vi "Adquisicion Sonido Continuo pruebas.vi"() -> ()   [LabVIEW 2023]
uses:
  <vilib>/sound2/lvsound2.llb/Sound Data Format.ctl
  <vilib>/sound2/lvsound2.llb/Sampling Mode.ctl
  <vilib>/sound2/lvsound2.llb/Sound Input Read (DBL).vi
  <vilib>/Analysis/3filter.llb/Butterworth Filter (DBL).vi
  <vilib>/measure/mamon.llb/Waveform Peak Detection for 1 Chan.vi
  <vilib>/measure/maspectr.llb/FFT Power Spectrum and PSD for 1 Chan.vi
  <vilib>/Waveform/DWDTOps.llb/DWDT Analog to Digital.vi
  <vilib>/express/express analysis/Spectral/Block/exnSpectralBlock spectral measurements power poly.vi
  <vilib>/express/express analysis/Spectral/Block/exnSpectralBlock spectral measurements power array WFM.vi
  <vilib>/express/express analysis/Spectral/XNode/ExpressSpectralMeasurementsBlockNode.xnode
  <vilib>/measure/NI_MABase.lvlib
  <vilib>/measure/NI_MAPro.lvlib
  <vilib>/Analysis/NI_AALBase.lvlib
panel:
  in  "Phase 6":dbl(knob) scale=0.0..360.0
  in  "alta frec filtrada 2":T1(ring)
  in  "phase 5":dbl(knob) scale=0.0..360.0
  in  "baja frec filtrada 2":T1(ring)
  in  "frequency 2":dbl=10.0 format="%0.2p"
  in  "frequency":dbl=10.0 format="%0.2p"
  out "# found":i32
  in  "peaks/valleys":u16(ring) items=["Peaks", "Valleys"]
  out "Lissajous 2":cluster{"Array":dbl[], "Array":dbl[]}(graph)
  in  "señal alta frec filtrada":T1(ring)
  in  "phase 4":dbl format="%.2p"
  in  "phase 3":dbl
  in  "señal baja frec filtrada":T1(ring)
  in  "alpha":dbl
  in  "stop 2":bool
  out "Lissajous":cluster{"Array":dbl[], "Array":dbl[]}[](graph)
  in  "señal alta frec":T1(ring)
  in  "phase 2":dbl format="%.2p"
  in  "Señal baja frec":T1(ring)
  in  "phase":dbl
  out "Max banda 2":i32
  out "Max banda 1":i32
  out "Tamaño banda 2":i32
  out "Plano Y":dbl[](array[numeric])
  out "Tamaño banda 1":i32
  out "Plano X":dbl[](array[numeric])
  in  "banda 2":dbl
  in  "banda 1":dbl
  out "Tamaño Señal":i32
  out "Espectro Señal":cluster{"f0":dbl, "df":dbl, "magnitude":dbl[]}[](graph)
  in  "stop":bool
  in  "Tiempo de refresco":dbl
  out "Señal Adquirida":waveform(dbl)[](graph)
  # "Señal sin Filtrado"
  # "Señal Filtrada"
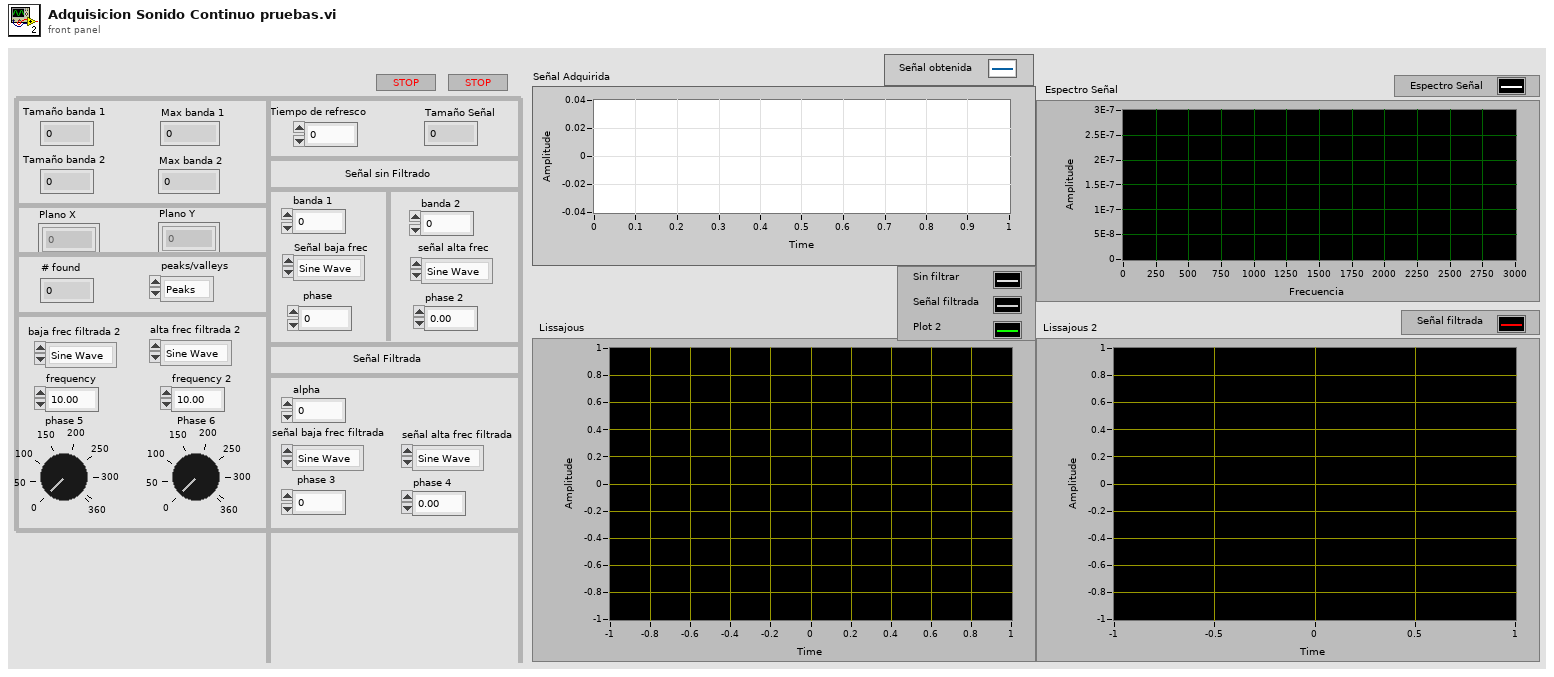
[diagram p1: front panel]
types:
  T1 = enum16{"Sine Wave", "Triangle Wave", "Square Wave", "Sawtooth Wave"}
  T2 = typedef "Sampling Mode.ctl" = i32
  T3 = typedef "Sound Data Format.ctl" = cluster{"sample rate (S/s)":dbl, "number of channels":i32, "bits per sample":i32}
  T4 = typedef "Sound Input Task ID.ctl" = u32
  T5 = cluster{"averaging mode":u16, "weighting mode":u16, "number of averages":u32}
  T6 = cluster{"dB On (F)":bool, "unwrap phase (F)":bool, "convert to degree (F)":bool}
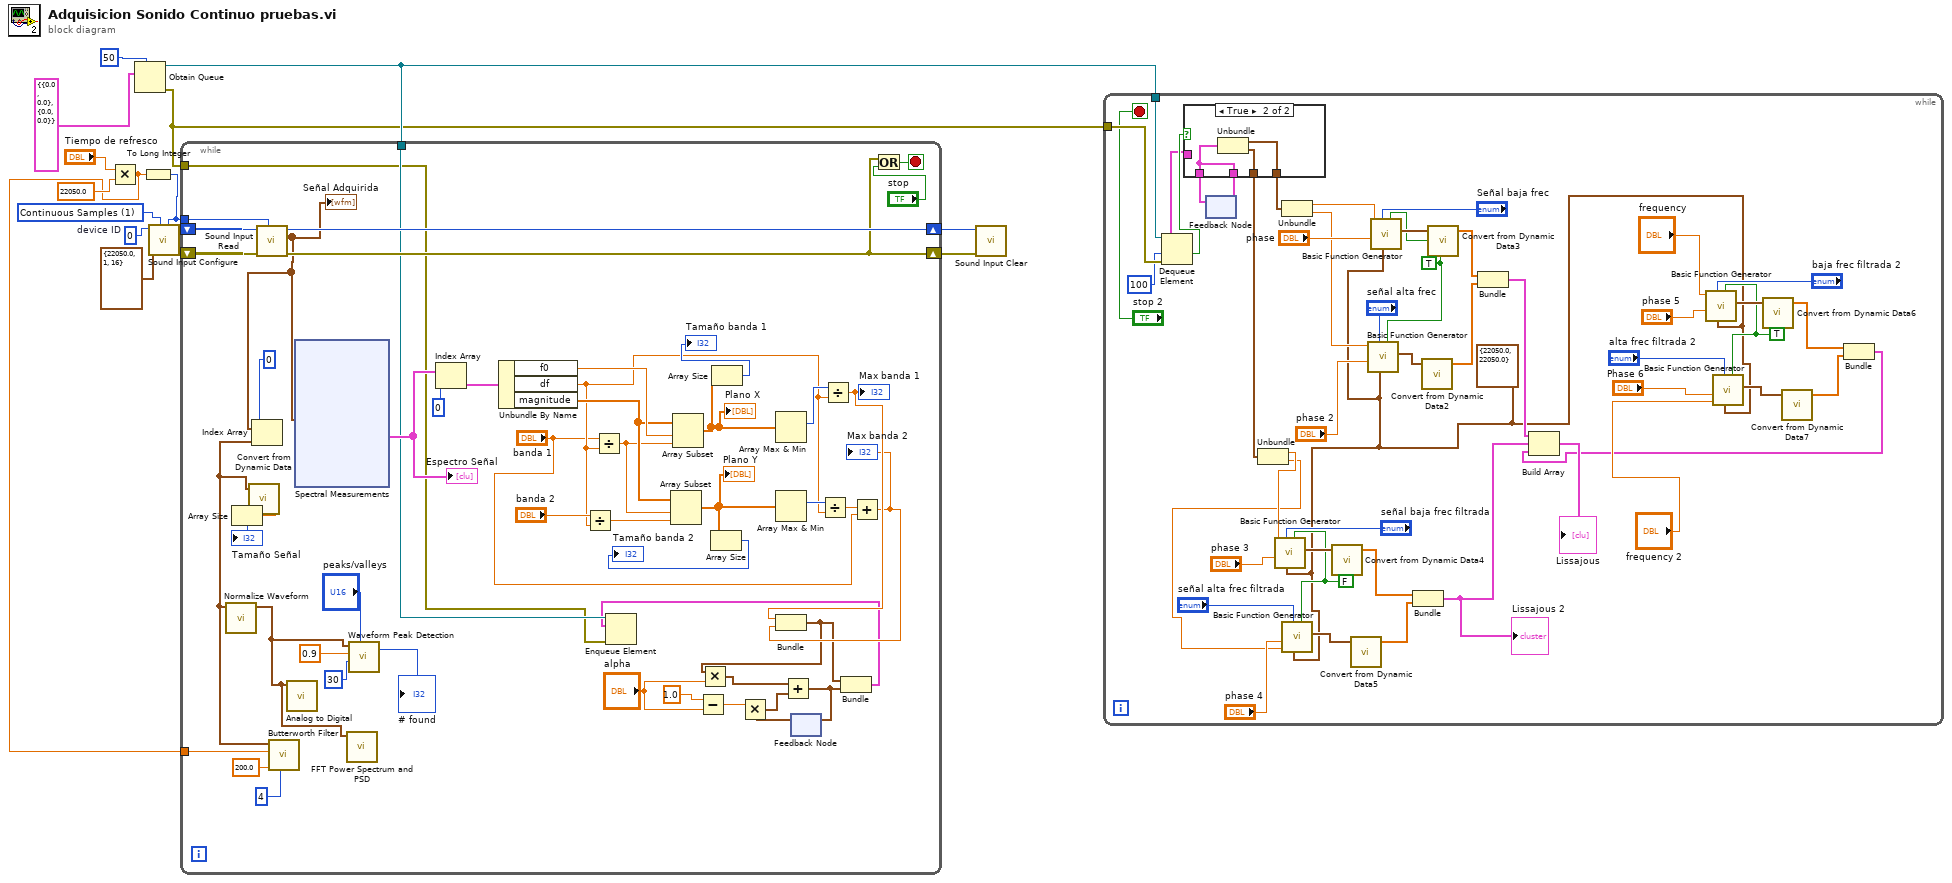
[diagram p0: block diagram]
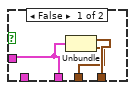
[diagram p2: hidden frame]
diagram:
  w11 = u32 0  # device ID
  w14 = T2 1 items=["Finite Samples", "Continuous Samples"] ("sample mode")
  n1 = Multiply(x="Tiempo de refresco", y=22050.0 ("number of samples/ch")) -> (x*y=w1:dbl)
  n2 = Obtain Queue(max queue size (-1, unlimited)=50, element data type=cluster{cluster{dbl, dbl}, cluster{dbl, dbl}} {{0.0, 0.0}, {0.0, 0.0}} ("output cluster")) -> (queue out=w5:refnum<queue>, error out=w4:errorcluster)  [unwired: 3 in, 1 out]
  n3 = To Long Integer(number=w1) -> (32bit integer=w7:i32)
  n4 = call <vilib>:"Sound Input Configure.vi"("number of samples/ch"=w7, "sample mode"=w14, "sound format"=T3 {"sample rate (S/s)"=22050.0, "number of channels"=1, "bits per sample"=16}, "device ID"=w11) -> ("error out"=w12:errorcluster, "task ID"=w13:T4)  [unwired: 6 in]
  n5 = while {
    tunnel: w7 -> [w26]
    shift-right: [w62] -> w9
    shift-left: w13 -> [w65]
    shift-right: [w61] -> w8
    shift-left: w12 -> [w64]
    tunnel: w5 -> [w41]
    tunnel: w4 -> [w40]
    tunnel: w1 -> [w19]
    stop <- w63 stop-if-true
    n6 = call-poly <vilib>:"Sound Input Read.vi"("number of samples/ch"=w26, "error in (no error)"=w64, "task ID"=w65) -> ("error out"=w61:errorcluster, "data"=w27:waveform(dbl)[], "task ID out"=w62:T4)  [unwired: 6 in]
    "Señal Adquirida" <- w27
    n7 = Index Array(array=w27, index=0) -> (element=w20:waveform(dbl))
    n8 = call <vilib>:"Normalize Waveform.vi"("waveform in"=w20) -> ("normalized waveform"=w16:waveform(dbl))  [unwired: 7 in, 3 out]
    n9 = call "Convert from Dynamic Data"("Dynamic Data Type"=w20) -> ("Array"=w56:dbl[])  [unwired: 3 in]
    n10 = Array Size(array=w56) -> (size(s)=→"Tamaño Señal":i32)
    n11 = call-poly <vilib>:"Butterworth Filter.vi"("order"=4, "low cutoff freq: fl"=200.0, "sampling freq: fs"=w19, "X"=w20) -> ()  [unwired: 4 in, 2 out]
    n12 = call-poly <vilib>:"Analog to Digital.vi"("analog waveform"=w16) -> ()  [unwired: 7 in, 4 out]
    n13 = xnode "Spectral Measurements"("Signals"=w27) -> ("Power Spectrum"=w58:cluster{"f0":dbl, "df":dbl, "magnitude":dbl[]}[])  [unwired: 1 in, 1 out]
    "Espectro Señal" <- w58
    n14 = call-poly <vilib>:"FFT Power Spectrum and PSD.vi"("time signal"=w16) -> ()  [unwired: 7 in, 4 out]
    n15 = call-poly <vilib>:"Waveform Peak Detection.vi"("peaks/valleys"="peaks/valleys", "width"=30, "threshold"=0.9, "Signal In"=w16) -> ("# found"=→"# found":i32)  [unwired: 3 in, 4 out]
    n16 = Index Array(array=w58, index=0) -> (element=w57:cluster{"f0":dbl, "df":dbl, "magnitude":dbl[]})
    n17 = Unbundle By Name(w57) -> ("f0"=w54:dbl, "df"=w42:dbl, "magnitude"=w51:dbl[])
    n18 = Divide(x="banda 2", y=w42) -> (x/y=w52:dbl)
    n19 = Divide(x="banda 1", y=w42) -> (x/y=w47:dbl)
    n20 = Array Subset(array=w51, index=w47, length=w52) -> (w46:dbl[])
    "Plano Y" <- w46
    n21 = Array Subset(array=w51, index=w54, length=w47) -> (w48:dbl[])
    "Plano X" <- w48
    n22 = Subtract(x=1.0, y="alpha") -> (x-y=w34:dbl)
    n23 = Array Size(array=w46) -> (size(s)=→"Tamaño banda 2":i32)
    n24 = Array Size(array=w48) -> (size(s)=→"Tamaño banda 1":i32)
    n25 = Array Max & Min(array=w48) -> (max index (indices)=w45:i32)  [unwired: 3 out]
    n26 = Array Max & Min(array=w46) -> (max index (indices)=w44:i32)  [unwired: 3 out]
    n27 = feedback #1() -> (w31:cluster{dbl, dbl})  [unwired: 1 in]
    n28 = Multiply(x=w34, y=w31) -> (x*y=w33:cluster{dbl, dbl})
    n29 = Divide(x=w44, y=w42) -> (x/y=w43:dbl)
    n30 = Divide(x=w45, y=w42) -> (x/y=w38:dbl)
    "Max banda 1" <- w38
    n31 = Add(x=w43, y="banda 1") -> (x+y=w37:dbl)
    "Max banda 2" <- w37
    n32 = Bundle(w38, w37) -> (w30:cluster{dbl, dbl})  [unwired: 1 in]
    n33 = Multiply(x=w30, y="alpha") -> (x*y=w32:cluster{dbl, dbl})
    n34 = Add(x=w32, y=w33) -> (x+y=w29:cluster{dbl, dbl})
    n35 = feedback-in #1(w29) -> ()
    n36 = Bundle(w30, w29) -> (w28:cluster{cluster{dbl, dbl}, cluster{dbl, dbl}})  [unwired: 1 in]
    n37 = Enqueue Element(queue=w41, element=w28, error in (no error)=w40) -> ()  [unwired: 4 out]
    n38 = Or(x=w61, y="stop") -> (x .or. y?=w63:bool)
  }
  n39 = call <vilib>:"Sound Input Clear.vi"("error in (no error)"=w8, "task ID"=w9) -> ()  [unwired: 9 in, 1 out]
  n40 = while {
    tunnel: w5 -> [w114]
    tunnel: w4 -> [w113]
    stop <- "stop 2" stop-if-true
    w80 = TRUE ("reset signal")
    w90 = TRUE ("reset signal")
    w92 = FALSE ("reset signal")
    w79 = cluster{"Fs":dbl, "#s":dbl} {"Fs"=22050.0, "#s"=22050.0} ("sampling info")
    n41 = Dequeue Element(queue=w114, timeout in ms (-1)=100, error in (no error)=w113) -> (element=w95:cluster{cluster{dbl, dbl}, cluster{dbl, dbl}}, timed out?=w99:bool)  [unwired: 2 out]
    n42 = feedback #2() -> (w96:cluster{cluster{dbl, dbl}, cluster{dbl, dbl}})  [unwired: 1 in]
    n43 = case shown="True" w99 {
      tunnel: [w125 w128] -> w98
      tunnel: [w124 w127] -> w97
      tunnel: w96 -> [_ w126]
      tunnel: w95 -> [w123 _]
      tunnel: [w123 w126] -> w94
      frame False {
        n44 = Unbundle(w123) -> (w125:cluster{dbl, dbl}, w124:cluster{dbl, dbl})
      }
      frame True {
        n45 = Unbundle(w126) -> (w128:cluster{dbl, dbl}, w127:cluster{dbl, dbl})
      }
    }
    n46 = feedback-in #2(w94) -> ()
    n47 = Unbundle(w97) -> (w89:dbl, w88:dbl)
    n48 = call <vilib>:"Basic Function Generator.vi"("reset signal"=w92, "sampling info"=w79, "signal type"="señal baja frec filtrada", "phase"="phase 3", "frequency"=w89) -> ("signal out"=w110:waveform(dbl))  [unwired: 4 in, 2 out]
    n49 = Unbundle(w98) -> (w111:dbl, w102:dbl)
    n50 = call <vilib>:"Basic Function Generator.vi"("reset signal"=w92, "sampling info"=w79, "signal type"="señal alta frec filtrada", "phase"="phase 4", "frequency"=w88) -> ("signal out"=w107:waveform(dbl))  [unwired: 4 in, 2 out]
    n51 = call "Convert from Dynamic Data4"("Dynamic Data Type"=w110) -> ("Array"=w105:dbl[])  [unwired: 3 in]
    n52 = call "Convert from Dynamic Data5"("Dynamic Data Type"=w107) -> ("Array"=w93:dbl[])  [unwired: 3 in]
    n53 = call <vilib>:"Basic Function Generator.vi"("reset signal"=w90, "sampling info"=w79, "signal type"="señal alta frec", "phase"="phase 2", "frequency"=w102) -> ("signal out"=w119:waveform(dbl))  [unwired: 4 in, 2 out]
    n54 = call <vilib>:"Basic Function Generator.vi"("reset signal"=w90, "sampling info"=w79, "signal type"="Señal baja frec", "phase"="phase", "frequency"=w111) -> ("signal out"=w120:waveform(dbl))  [unwired: 4 in, 2 out]
    n55 = Bundle("Array"=w105, "Array"=w93) -> (w91:cluster{"Array":dbl[], "Array":dbl[]})  [unwired: 1 in]
    "Lissajous 2" <- w91
    n56 = call "Convert from Dynamic Data2"("Dynamic Data Type"=w119) -> ("Array"=w121:dbl[])  [unwired: 3 in]
    n57 = call "Convert from Dynamic Data3"("Dynamic Data Type"=w120) -> ("Array"=w122:dbl[])  [unwired: 3 in]
    n58 = Bundle("Array"=w122, "Array"=w121) -> (w104:cluster{"Array":dbl[], "Array":dbl[]})  [unwired: 1 in]
    n59 = call <vilib>:"Basic Function Generator.vi"("reset signal"=w80, "sampling info"=w79, "signal type"="baja frec filtrada 2", "phase"="phase 5", "frequency"="frequency") -> ("signal out"=w87:waveform(dbl))  [unwired: 4 in, 2 out]
    n60 = call <vilib>:"Basic Function Generator.vi"("reset signal"=w80, "sampling info"=w79, "signal type"="alta frec filtrada 2", "phase"="Phase 6", "frequency"="frequency 2") -> ("signal out"=w84:waveform(dbl))  [unwired: 4 in, 2 out]
    n61 = call "Convert from Dynamic Data6"("Dynamic Data Type"=w87) -> ("Array"=w83:dbl[])  [unwired: 3 in]
    n62 = call "Convert from Dynamic Data7"("Dynamic Data Type"=w84) -> ("Array"=w81:dbl[])  [unwired: 3 in]
    n63 = Bundle("Array"=w83, "Array"=w81) -> (w76:cluster{"Array":dbl[], "Array":dbl[]})  [unwired: 1 in]
    n64 = Build Array(w104, w91, w76) -> (→"Lissajous":cluster{"Array":dbl[], "Array":dbl[]}[])
  }
